vi "Write Static Overlays.vi"(8 "error in (no error)":errorcluster, 10 "Static Overlays":refnum<class "Static Overlay.lvclass">[](array[class]), 11 "HIJ Vision Application in":refnum<class "HIJ Vision Application.lvclass">) -> (0 "error out":errorcluster, 3 "HIJ Vision Application out":refnum<class "HIJ Vision Application.lvclass">)   [LabVIEW 2020, in "HIJ Vision Application.lvlib" / "HIJ Vision Application.lvclass"]
uses:
  HIJ Vision Application.lvclass
  Analyze/Results and Overlays/Static Overlay/Static Overlay.lvclass
  HIJ Vision Application.lvclass/HIJ Vision Application.ctl
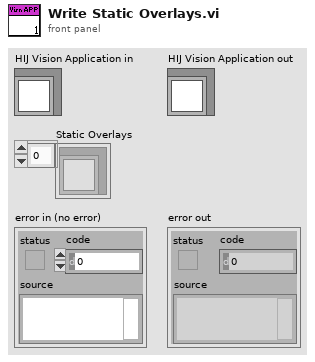
[diagram p1: front panel]
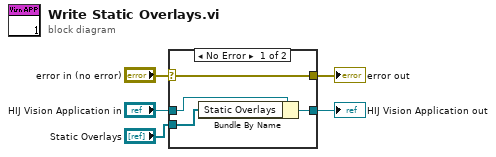
[diagram p0: block diagram]
diagram:
  n1 = case shown="No Error" "error in (no error)" {
    selector: "error in (no error)" -> [w6 w11]
    tunnel: [w6 w11] -> w4
    tunnel: [w8 w10] -> w2
    tunnel: "HIJ Vision Application in" -> [w9 w10]
    tunnel: "Static Overlays" -> [w7 _]
    frame No Error {
      n2 = Bundle By Name(cluster=w9, "Static Overlays"=w7) -> (w8:refnum<class "HIJ Vision Application.lvclass">)
    }
    frame Error {
    }
  }
  "error out" <- w4
  "HIJ Vision Application out" <- w2
